vi "closeShutter.vi"   [LabVIEW 2014]
doc: "Newport Motion Controler\nClose Shutter communication port\n\nAndré Romero - 2020\nandretec@ifsc.usp.br"
uses:
  Global Shutter.vi
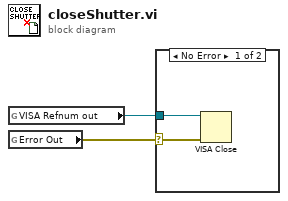
[diagram p0: block diagram]
diagram:
  n1 = global read "Global Shutter.vi" "VISA Refnum out"() -> (w2:refnum<visa-resource-name>)
  n2 = global read "Global Shutter.vi" "Error Out"() -> (w1:errorcluster)
  n3 = case shown="No Error" w1 {
    selector: w1 -> [w3 _]
    tunnel: w2 -> [w4 _]
    frame No Error {
      n4 = VISA Close(VISA resource name=w4, error in (no error)=w3) -> ()  [unwired: 1 out]
    }
    frame Error {
    }
  }
